vi "9自相关子程序.vi"(7 "time signal":waveform(dbl) caption="时间信号") -> (3 "波形图":waveform(dbl)(graph))   [LabVIEW 2017]
uses:
  <vilib>/Analysis/NI_AALPro.lvlib
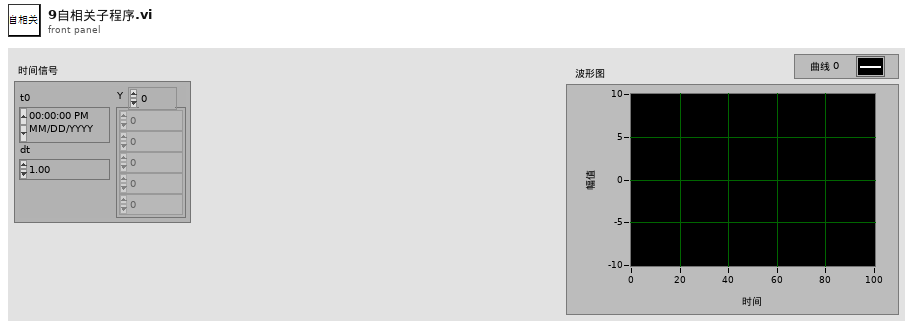
[diagram p1: front panel]
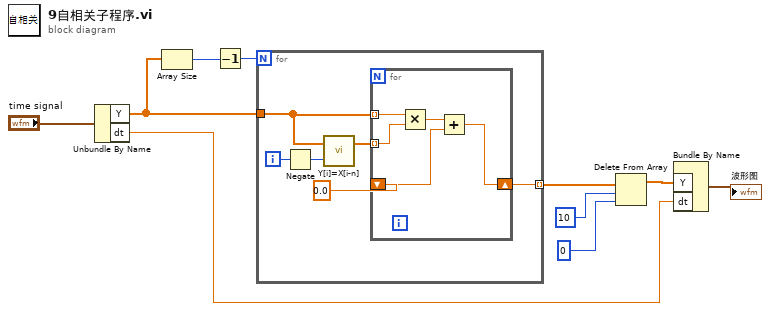
[diagram p0: block diagram]
diagram:
  n1 = Unbundle By Name("time signal") -> ("Y"=w10:dbl[], "dt"=w2:dbl)
  n2 = Array Size(array=w10) -> (size(s)=w3:i32)
  n3 = Decrement(x=w3) -> (x-1=w9:i32)
  n4 = for {
    N: w9 -> [_]
    tunnel: w10 -> [w15]
    tunnel: [w13] -> w1 mode=indexing
    i -> [w12]
    n5 = Negate(x=w12) -> (-x=w11:i32)
    n6 = call <vilib>:"Y[i]=X[i-n].vi"("shifts: n"=w11, "Input Array"=w15) -> ("Shifted Array"=w16:dbl[])  [unwired: 1 out]
    n7 = for {
      tunnel: w16 -> [w20] mode=indexing
      tunnel: w15 -> [w21] mode=indexing
      shift-right: [w17] -> w13
      shift-left: 0.0 -> [w18]
      n8 = Multiply(x=w21, y=w20) -> (x*y=w19:dbl)
      n9 = Add(x=w19, y=w18) -> (x+y=w17:dbl)
    }
  }
  n10 = Delete From Array(array=w1, length=10 ("长度"), index=0 ("索引")) -> (array with subset deleted=w6:dbl[])  [unwired: 1 out]
  n11 = Bundle By Name("Y"=w6, "dt"=w2) -> (→"波形图":waveform(dbl))  [unwired: 1 in]
